vi "Read Attributes.vi"(11 "WebSocket Data Msg":refnum<class "WebSocket Service Enqueuer Msg.lvclass">) -> (2 "Payload":cluster{"Data":string})   [LabVIEW 2016, in "WebSocket Actor.lvlib" / "WebSocket Service Enqueuer Msg.lvclass"]
uses:
  WebSocket Service Enqueuer Msg.lvclass
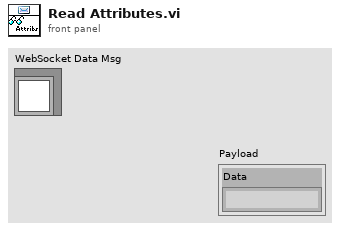
[diagram p1: front panel]
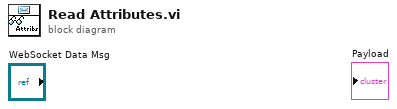
[diagram p0: block diagram]
diagram:
